vi "Arrange messages.vi"(11 "Array in":T1(array[cluster]) {"DATA[0]" format="%.0x"}) -> (3 "Array out":T1(array[cluster]))   [LabVIEW 2023]
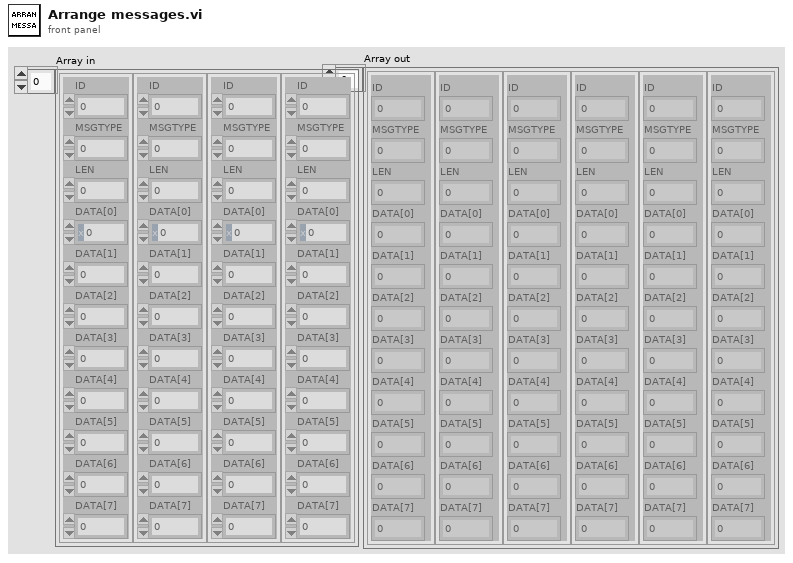
[diagram p1: front panel]
types:
  T1 = cluster{"ID":u32, "MSGTYPE":u8, "LEN":u8, "DATA[0]":u8, "DATA[1]":u8, "DATA[2]":u8, "DATA[3]":u8, "DATA[4]":u8, "DATA[5]":u8, "DATA[6]":u8, "DATA[7]":u8}[]
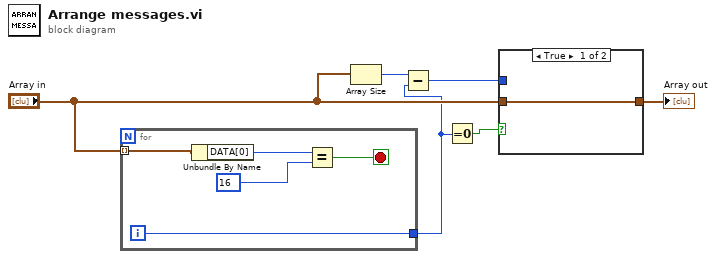
[diagram p0: block diagram]
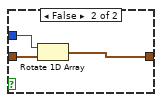
[diagram p2: hidden frame]
diagram:
  n1 = for {
    tunnel: "Array in" -> [w11] mode=indexing
    tunnel: [w7] -> w2
    i -> [w7]
    stop <- w8 stop-if-true
    n2 = Unbundle By Name(w11) -> ("DATA[0]"=w10:u8)
    n3 = Equal?(x=w10, y=u8 16) -> (x = y?=w8:bool)
  }
  n4 = Array Size(array="Array in") -> (size(s)=w4:i32)
  n5 = Subtract(x=w4, y=w2) -> (x-y=w3:i32)
  n6 = Equal To 0?(x=w2) -> (x = 0?=w1:bool)
  n7 = case shown="True" w1 {
    tunnel: [w12 w15] -> w6
    tunnel: "Array in" -> [w12 w14]
    tunnel: w3 -> [_ w13]
    frame True {
    }
    frame False {
      n8 = Rotate 1D Array(1:w14, 2:w13) -> (0:w15:T1)
    }
  }
  "Array out" <- w6
